vi "Write_IMAXdx-Attributes.vi"(3 "error in":errorcluster, 4 "IMAQdx-Defaults":string="CameraAttributes::AnalogControl::GainSelector ,Enum ,1,1, 0  \nCameraAttributes::AcquisitionControl::ExposureAuto ,Enum ,1,1, 0  ", 5 "Session In":T3) -> (0 "error out":errorcluster, 2 "Session Out":T3)   [LabVIEW 2011]
uses:
  <vilib>/userDefined/High Color/IMAQdx.ctl
  <vilib>/vision/driver/IMAQdx.llb/IMAQdx Attribute Type.ctl
  C:/Program Files/National Instruments/LabVIEW 2011/resource/objmgr/imaqdx.rc
  <vilib>/vision/driver/NI_Vision_Acquisition_Software.lvlib
panel:
  out "Attribute Information 2":T2
  # "! Space nach name und type vor komma\nName, \nType[U32,I64,DBL,String,Enum,Bool,Command], \nRead, \nWrite[0,1], \nValue"
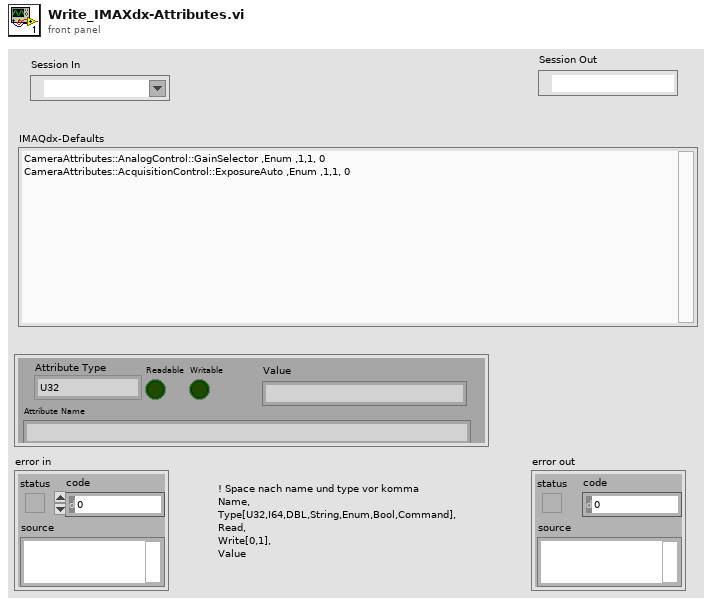
[diagram p1: front panel]
types:
  T1 = typedef "NI_Vision_Acquisition_Software.lvlib/IMAQdx Attribute Type.ctl" = enum32{"U32", "I64", "DBL", "String", "Enum", "Bool", "Command"}
  T2 = cluster{"Attribute Type":T1, "Readable":bool, "Writable":bool, "Attribute Name":string, "Value":string}
  T3 = typedef "IMAQdx.ctl" = refnum<k21>
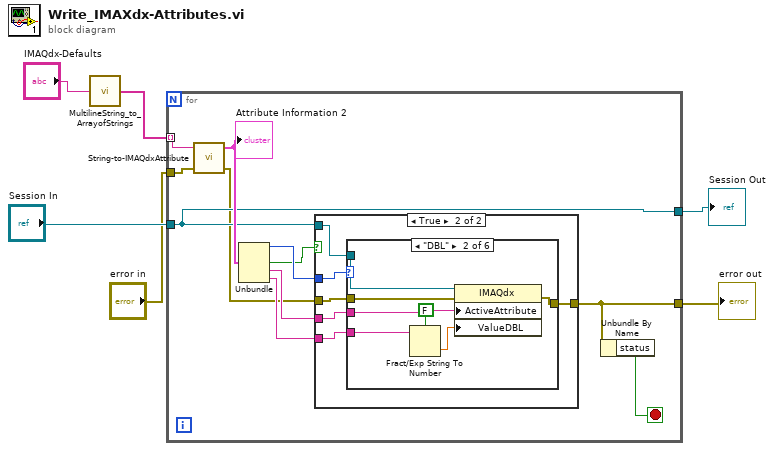
[diagram p0: block diagram]
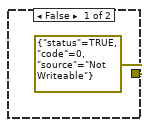
[diagram p2: hidden frame]
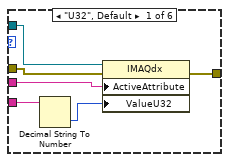
[diagram p3: hidden frame]
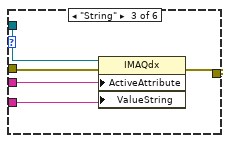
[diagram p4: hidden frame]
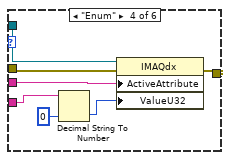
[diagram p5: hidden frame]
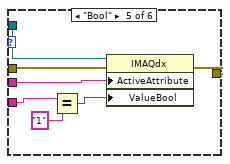
[diagram p6: hidden frame]
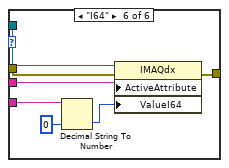
[diagram p7: hidden frame]
diagram:
  n1 = call "MultilineString_to_ArrayofStrings.vi"("String 1"="IMAQdx-Defaults") -> ("String Array"=w5:string[])  [unwired: 1 in]
  n2 = for {
    tunnel: w5 -> [w17] mode=indexing
    tunnel: "Session In" -> [w15]
    tunnel: [w15] -> w3
    tunnel: "error in" -> [w9]
    tunnel: [w7] -> w1
    stop <- w8 stop-if-true
    n3 = call "String-to-IMAQdxAttribute.vi"("error in"=w9, "IMAQdx-string"=w17) -> ("error out"=w10:errorcluster, "Attribute Information 2"=w16:T2)  [unwired: 1 in, 1 out]
    "Attribute Information 2" <- w16
    n4 = Unbundle(w16) -> ("Attribute Type"=w13:T1, "Writable"=w12:bool, "Attribute Name"=w14:string, "Value"=w11:string)  [unwired: 1 out]
    n5 = case shown="True" w12 {
      tunnel: w14 -> [_ w24]
      tunnel: w15 -> [_ w23]
      tunnel: w13 -> [_ w22]
      tunnel: w11 -> [_ w21]
      tunnel: [errorcluster {"status"=TRUE, "code"=0, "source"="Not Writeable"} ("error out") w20] -> w7
      tunnel: w10 -> [_ w19]
      frame False {
      }
      frame True {
        n6 = case shown="\"DBL\"" w22 {
          tunnel: w24 -> [w30 w37 w42 w49 w56 w63]
          tunnel: w23 -> [w29 w36 w41 w48 w55 w62]
          tunnel: w21 -> [w28 w34 w40 w47 w54 w61]
          tunnel: [w26 w35 w39 w46 w51 w58] -> w20
          tunnel: w19 -> [w25 w31 w38 w43 w50 w57]
          frame "U32", Default {
            n7 = Decimal String To Number(string=w28) -> (number=w27:i32)  [unwired: 2 in, 1 out]
            n8 = property class="IMAQdx"(reference=w29, error in=w25, "ActiveAttribute"=w30, "ValueU32"=w27) -> (error out=w26:errorcluster)  [unwired: 1 out]
          }
          frame "DBL" {
            n9 = Fract/Exp String To Number(use system decimal point (T)=FALSE, string=w34) -> (number=w32:dbl)  [unwired: 2 in, 1 out]
            n10 = property class="IMAQdx"(reference=w36, error in=w31, "ActiveAttribute"=w37, "ValueDBL"=w32) -> (error out=w35:errorcluster)  [unwired: 1 out]
          }
          frame "String" {
            n11 = property class="IMAQdx"(reference=w41, error in=w38, "ActiveAttribute"=w42, "ValueString"=w40) -> (error out=w39:errorcluster)  [unwired: 1 out]
          }
          frame "Enum" {
            n12 = Decimal String To Number(string=w47, default (0L)=0 ("default (0 I32)")) -> (number=w45:i32)  [unwired: 1 in, 1 out]
            n13 = property class="IMAQdx"(reference=w48, error in=w43, "ActiveAttribute"=w49, "ValueU32"=w45) -> (error out=w46:errorcluster)  [unwired: 1 out]
          }
          frame "Bool" {
            n14 = Equal?(x=w54, y="1") -> (x = y?=w52:bool)
            n15 = property class="IMAQdx"(reference=w55, error in=w50, "ActiveAttribute"=w56, "ValueBool"=w52) -> (error out=w51:errorcluster)  [unwired: 1 out]
          }
          frame "I64" {
            n16 = Decimal String To Number(string=w61, default (0L)=i64 0 ("default (0 I32)")) -> (number=w59:i64)  [unwired: 1 in, 1 out]
            n17 = property class="IMAQdx"(reference=w62, error in=w57, "ActiveAttribute"=w63, "ValueI64"=w59) -> (error out=w58:errorcluster)  [unwired: 1 out]
          }
        }
      }
    }
    n18 = Unbundle By Name(w7) -> ("status"=w8:bool)
  }
  "Session Out" <- w3
  "error out" <- w1
